vi "LaserLineDetection_AVI_Intensity_main.vi"() -> ()   [LabVIEW 2013]
doc: "This example shows how to open, read, and display an AVI file in NI Vision. The VI reads the frames per second property and plays the images back at the rate specified by the AVI file."
panel:
  out "Perpendicular Distance":dbl
  in  "F = Gauss S\nT = Gauss ES":bool
  out "Laser Detected":bool
  in  "index (row)":i32
  out "Incident Angle":dbl
  in  "F = I_max\nT = Gauss":bool
  out "Distance":dbl
  in  "milliseconds to wait":u32=100
  out "Intensity":cluster{u8[], i32[]}[](graph)
  in  "Pause":bool
  out "Seconds to Wait":dbl
  in  "Progress Bar":u32(slide) max=191 scale=-1.0..191.0
  in  "Stop":bool
  out "Source":T1(plugin-control)
  # "1m = 850"
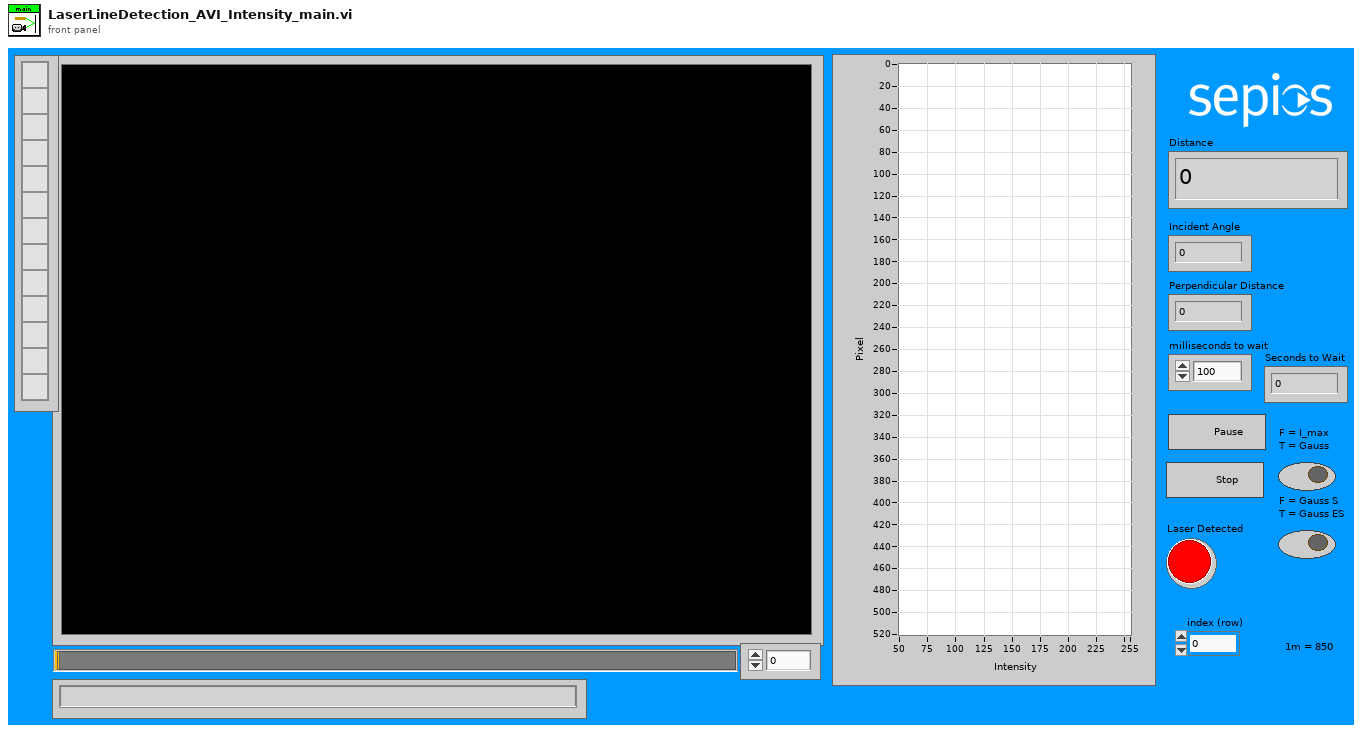
[diagram p1: front panel]
types:
  T1 = typedef "IMAQ Image.ctl" = refnum<image>
  T2 = typedef "IMAQ AVI2 Refnum.ctl" = refnum<k20>
  T3 = typedef "Image Type" = u32
  T4 = cluster{"Width":u32, "Height":u32, "Frames Per Second":u32, "Codec":string, "Has Data":bool}
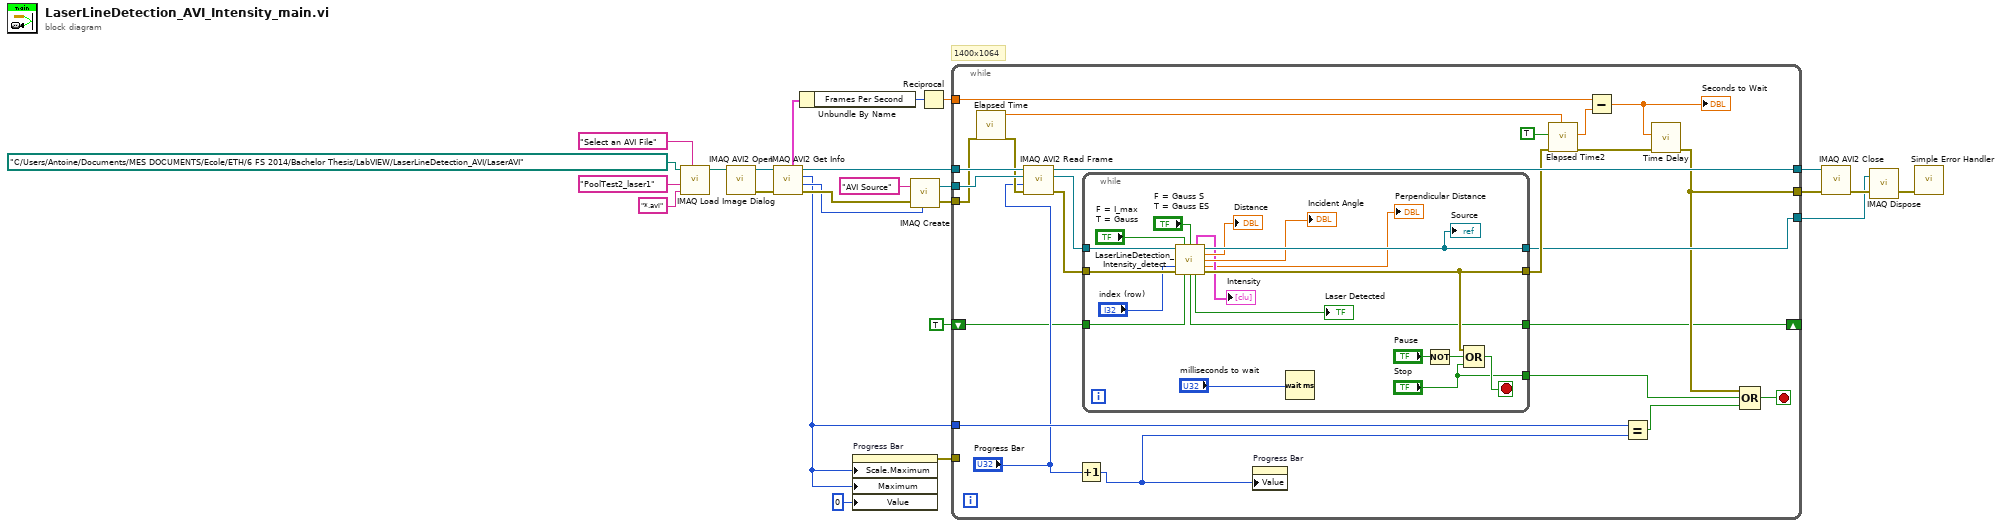
[diagram p0: block diagram]
diagram:
  # "1400x1064"
  n1 = call "IMAQ Load Image Dialog"("Prompt"="Select an AVI File" ("prompt"), "Pattern"="*.avi", "Default Name"="PoolTest2_laser1", "Start Path"=path "C:/Users/Antoine/Documents/MES DOCUMENTS/Ecole/ETH/6 FS 2014/Bachelor Thesis/LabVIEW/LaserLineDetection_AVI/LaserAVI") -> ("Path"=w11:path)  [unwired: 5 in, 2 out]
  n2 = call "IMAQ AVI2 Open"("AVI File Path"=w11) -> ("error out"=w23:errorcluster, "AVI Refnum"=w22:T2)  [unwired: 2 in, 7 out]
  n3 = call "IMAQ AVI2 Get Info"("error in (no error)"=w23, "AVI Refnum"=w22) -> ("error out"=w19:errorcluster, "Image Type"=w15:T3, "Number of Frames"=w5:u32, "AVI Refnum (duplicate)"=w17:T2, "Frame Data"=w24:T4)  [unwired: 5 out]
  n4 = Unbundle By Name(w24) -> ("Frames Per Second"=w14:u32)
  n5 = property on="Progress Bar" class="Slide (strict)"("Scale.Maximum"=w5, "Maximum"=w5, "Value"=u32 0 ("Progress Bar")) -> (error out=w9:errorcluster)  [unwired: 2 in, 1 out]
  n6 = call "IMAQ Create"("Image Name"="AVI Source", "Image Type"=w15, "error in (no error)"=w19) -> ("New Image"=w18:T1, "error out"=w2:errorcluster)  [unwired: 1 in, 1 out]
  n7 = Reciprocal(x=w14) -> (1/x=w13:dbl)
  n8 = while {
    tunnel: w18 -> [w48]
    tunnel: [w47] -> w20
    tunnel: [w33] -> w21
    tunnel: w2 -> [w46]
    tunnel: w17 -> [w49]
    tunnel: w13 -> [w44]
    tunnel: w9 -> [_]
    tunnel: [w35] -> w6
    tunnel: w5 -> [w34]
    shift-right: [w27] -> _
    shift-left: TRUE ("Laser Detected") -> [w26]
    stop <- w30 stop-if-true
    n9 = call "Elapsed Time"("error in (no error)"=w46) -> ("Present (s)"=w42:dbl, "error out"=w45:errorcluster)  [unwired: 11 in, 6 out]
    n10 = call "IMAQ AVI2 Read Frame"("error in (no error)"=w45, "Frame Number"="Progress Bar", "Image"=w48, "AVI Refnum"=w49) -> ("error out"=w37:errorcluster, "Image Out"=w38:T1, "AVI Refnum (duplicate)"=w47:T2)  [unwired: 5 out]
    n11 = Increment(x="Progress Bar") -> (x+1=w28:u32)
    n12 = while {
      tunnel: w38 -> [w61]
      tunnel: [w60] -> w35
      tunnel: w37 -> [w62]
      tunnel: [w63] -> w36
      tunnel: ["Stop"] -> w32
      tunnel: [w56] -> w27
      tunnel: w26 -> [w55]
      stop <- w67 stop-if-true
      n13 = call "LaserLineDetection_Intensity_detect.vi"("Source In"=w61, "F = I_max\nT = Gauss"="F = I_max\nT = Gauss", "F = Gauss S\nT = Gauss ES"="F = Gauss S\nT = Gauss ES", "index"="index (row)", "Error In"=w62, "Laser Detected Old"=w55) -> ("appended array"=→"Intensity":cluster{u8[], i32[]}[], "Source Out"=w60:T1, "Distance to Wall (m)"=→"Distance":dbl, "delta° (incident angle)"=→"Incident Angle":dbl, "Perpendicular Distance to Wall (m)"=→"Perpendicular Distance":dbl, "Laser Detected"=w56:bool, "Laser Detected Twice"=→"Laser Detected":bool, "Error Out"=w63:errorcluster)  [unwired: 2 in]
      "Source" <- w60
      n14 = Wait (ms)(milliseconds to wait="milliseconds to wait") -> ()  [unwired: 1 out]
      n15 = Not(x="Pause") -> (.not. x?=w66:bool)
      n16 = Compound Arithmetic op=OR(w63, w66, "Stop") -> (w67:bool)
    }
    n17 = property on="Progress Bar" class="Slide (strict)"("Value"=w28) -> ()  [unwired: 2 in, 2 out]
    n18 = call "Elapsed Time2"("Reset"=TRUE, "error in (no error)"=w36, "Set Start Time (s)"=w42) -> ("Elapsed Time (s)"=w40:dbl, "error out"=w39:errorcluster)  [unwired: 9 in, 6 out]
    n19 = Subtract(x=w44, y=w40) -> (x-y=w43:dbl)
    "Seconds to Wait" <- w43
    n20 = Equal?(x=w34, y=w28) -> (x = y?=w31:bool)
    n21 = call "Time Delay"("error in (no error)"=w39, "Delay Time (s)"=w43) -> ("error out"=w33:errorcluster)  [unwired: 9 in]
    n22 = Compound Arithmetic op=OR(w33, w32, w31) -> (w30:bool)
  }
  n23 = call "IMAQ AVI2 Close"("error in (no error)"=w21, "AVI Refnum"=w20) -> ("error out"=w16:errorcluster)  [unwired: 9 out]
  n24 = call "IMAQ Dispose"("Image"=w6, "error in (no error)"=w16) -> ("error out"=w3:errorcluster)  [unwired: 1 in, 3 out]
  n25 = call <vilib>:"Simple Error Handler.vi"("error in (no error)"=w3) -> ()  [unwired: 1 in, 8 out]
